vi "Async.Engine.Initialize.vi"(8 "error in (no error)":errorcluster, 10 "Processes":cluster{"VI":refnum<vi>, "Parameters":variant}[](array[cluster]), 11 "Custom Device Ref":T1 format="%.0x") -> (0 "error out":errorcluster, 3 "Async":refnum<class "VS Inline Async API.lvclass">)   [LabVIEW 2015, in "VS Inline Async API.lvlib" / "VS Inline Async API.lvclass"]
uses:
  VS Inline Async API.lvclass
  <vilib>/NI Veristand/Custom Device API/Custom Device Item Ref.ctl
  VS Inline Async API.lvclass/VS Inline Async API.ctl
  Error Handling Process/SubVIs/Error.GetError.vi
  <vilib>/Utility/error.llb/Error Cluster From Error Code.vi
  VS Inline Async API.lvlib
  _Data Access Engine/Data Access Engine/Data Access Engine.lvclass
  <vilib>/NI Veristand/Custom Device API/Custom Device API.lvlib
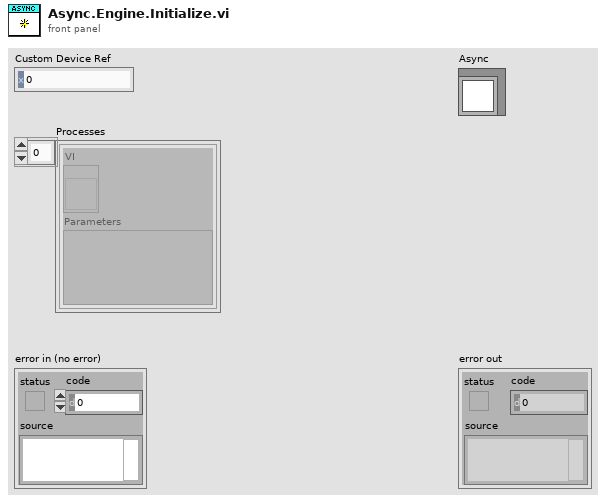
[diagram p1: front panel]
types:
  T1 = typedef "Custom Device API.lvlib/Custom Device Item Ref.ctl" = u64
  T2 = typedef "Custom Device API.lvlib/Custom Device Item Info.ctl" = cluster{"Name":string, "Is Channel":bool, "GUID":string, "Is Waveform":bool}
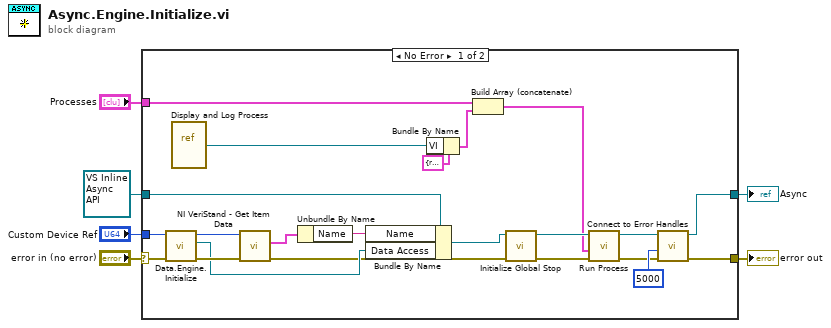
[diagram p0: block diagram]
diagram:
  n1 = case shown="No Error" "error in (no error)" {
    selector: "error in (no error)" -> [w15 w30]
    tunnel: [w24 w30] -> w5
    tunnel: [w22 w29] -> w3
    tunnel: refnum<class "VS Inline Async API.lvclass"> refnum ("Async in") -> [w27 w29]
    tunnel: "Processes" -> [w26 _]
    tunnel: "Custom Device Ref" -> [w14 _]
    frame No Error {
      n2 = call "Data.Engine.Initialize.vi"("error in"=w15, "Custom Device Ref"=w14) -> ("error out"=w13:errorcluster, "Data Access Engine"=w9:refnum<class "Data Access Engine.lvclass">, "Custom Device Ref"=w12:T1)  [unwired: 7 in]
      n3 = vi-ref "Display and Log Process.vi"() -> (w20:refnum<vi>)
      n4 = call <vilib>:"NI VeriStand - Get Item Data.vi"("error in (no error)"=w13, "Item Ref in"=w12) -> ("error out"=w8:errorcluster, "Item Info"=w11:T2)  [unwired: 6 in, 2 out]
      n5 = Unbundle By Name(w11) -> ("Name"=w10:string)
      n6 = Bundle By Name(cluster=w27, "Name"=w10, "Data Access"=w9) -> (w7:refnum<class "VS Inline Async API.lvclass">)
      n7 = Bundle By Name(cluster=cluster{"VI":refnum<vi>, "Parameters":variant} {"VI"=refnum, "Parameters"=variant} ("Process"), "VI"=w20) -> (w19:cluster{"VI":refnum<vi>, "Parameters":variant})
      n8 = Build Array (concatenate)(w26, w19) -> (w16:cluster{"VI":refnum<vi>, "Parameters":variant}[])
      n9 = call "Initialize Global Stop.vi"("error in (no error)"=w8, "Async in"=w7) -> ("error out"=w18:errorcluster, "Async out"=w17:refnum<class "VS Inline Async API.lvclass">)  [unwired: 8 in]
      n10 = call "Run Process.vi"("error in (no error)"=w18, "Processes"=w16, "Async in"=w17) -> ("error out"=w25:errorcluster, "Async out"=w23:refnum<class "VS Inline Async API.lvclass">)  [unwired: 7 in]
      n11 = call "Connect to Error Handles.vi"("error in"=w25, "Timeout (ms)"=u16 5000, "Async in"=w23) -> ("error out"=w24:errorcluster, "Async out"=w22:refnum<class "VS Inline Async API.lvclass">)  [unwired: 7 in]
    }
    frame Error {
    }
  }
  "error out" <- w5
  "Async" <- w3
